vi "Query.vi"(7 "IP":string="192.168.23.100", 8 "error in (no error)":errorcluster, 9 "PARAMETERS":string, 10 "PORT":dbl=1.0 min=1.0 max=4.0 step=1.0, 11 "MASTER":dbl=1.0 min=1.0 max=10.0 step=1.0) -> (0 "error out":errorcluster, 3 "JSON data":string)   [LabVIEW 2022 SP3]
uses:
  <vilib>/NI/Advanced HTTP Client/Session.lvclass
panel:
  # "Parameter Query"
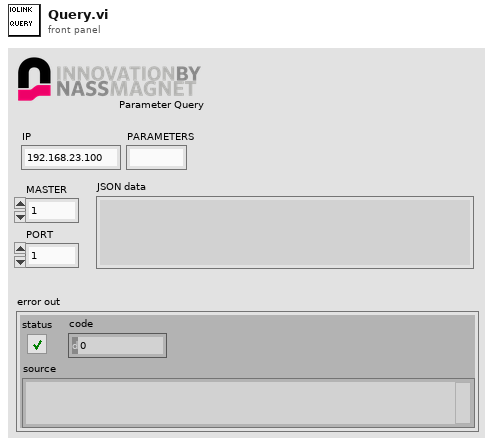
[diagram p1: front panel]
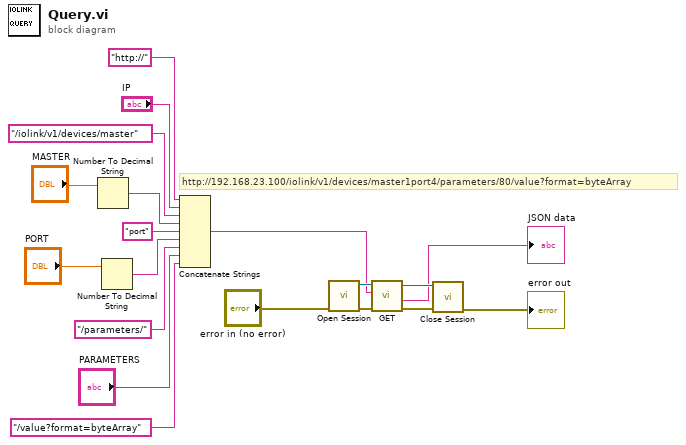
[diagram p0: block diagram]
diagram:
  # "http://192.168.23.100/iolink/v1/devices/master1port4/parameters/80/value?format=byteArray"
  n1 = Number To Decimal String(number="MASTER") -> (decimal integer string=w8:string)  [unwired: 1 in]
  n2 = Number To Decimal String(number="PORT") -> (decimal integer string=w5:string)  [unwired: 1 in]
  n3 = Concatenate Strings("http://" ("string"), "IP", "/iolink/v1/devices/master" ("string"), w8, "port" ("string"), w5, "/parameters/" ("string"), "PARAMETERS", "/value?format=byteArray" ("string")) -> (w9:string)
  n4 = call <vilib>:"Open Session.vi"("error in"="error in (no error)") -> ("error out"=w18:errorcluster, "session"=w19:refnum<class "Session.lvclass">)  [unwired: 9 in]
  n5 = call <vilib>:"GET.vi"("error in"=w18, "url"=w9, "session in"=w19) -> ("error out"=w3:errorcluster, "body"=→"JSON data":string, "session out"=w4:refnum<class "Session.lvclass">)  [unwired: 4 in, 2 out]
  n6 = call <vilib>:"Close Session.vi"("error in"=w3, "session"=w4) -> ("error out"=→"error out":errorcluster)  [unwired: 9 in]
